vi "ABR3-Initialize.vi"(0 "Params":T1={"CAP or ABR"=enum."ABR", "Stimulus"={"Ear"=enum."Left", "Waveform"=enum."TONE PIP", "Frequency (kHz)"="", "Rep rate (/sec)"=30.0, "Alternate Polarity"=FALSE, "WavFiles"="", "Level (dB SPL)"=30.0, "WavFolder"=path "", "Chirp"={"Type"=enum."AN latency-corrected", "Duration (ms)"=0.0, "Fmin (kHz)"=0.0, "Fmax (kHz)"=0.0, "precompensate"=FALSE}, "Noise"={"Seed"=0, "InvFilt"=FALSE, "AWeight"=FALSE, "afile"=path "", "Filter"={"Type"=enum."Lowpass", "CF (kHz)"=0.0, "BW (kHz)"=0.0, "Cascade"=FALSE, "Quadrature"=FALSE, "Scale Factor"=0.0, "Stages"=[], "Class"=enum."Elliptic", "Order"=0, "BWUnits"=enum."Linear"}}}, "Masker"={"Filter"={"Type"=enum."Lowpass", "CF (kHz)"=0.0, "BW (kHz)"=0.0, "Cascade"=FALSE, "Quadrature"=FALSE, "Scale Factor"=0.0, "Stages"=[], "Class"=enum."Elliptic", "Order"=0, "BWUnits"=enum."Linear"}, "Use masker"=FALSE, "Level"={"Level"=0.0, "Units"=enum."dB atten", "Max"=0.0, "Multiplier"=0.0, "Cal File"=path "", "Cal"={"Freq (Hz)"=[], "Mag (dB SPL)"=[], "Phase (deg)"=[]}}, "Audiogram Comp"=FALSE, "Audiogram File"=path "", "InvFilt"=FALSE}, "Sequence"={"Start (dB)"=20, "Stop (dB)"=80, "Step (dB)"=5, "Var"=enum."Signal", "Order"=enum."Sequential"}, "Controls"={"on"=FALSE, "value"=0.0, "spacing"=0}, "Response"={"Gain"=10000, "Averages"=512, "Window (ms)"=8.5, "Thr Fast Steps"=8.5, "AI Fs"=0.0}, "Hidden"={"AO Samp Rate Hz"=100000.0, "Duration (ms)"=5.0, "Ramp (ms)"=0.5, "Click width (us)"=0.0}} {"Response"."Thr Fast Steps" format="%.2f"; "Response"."Window (ms)" format="%.2f"; "Sequence"."Start (dB)" step=5}, 1 "State":T39, 2 "Resume":bool, 11 "error in (no error)":errorcluster, 12 "Analysis In":T12) -> (3 "Runtime":T37={"Ceiling"=0.0, "Threshold"=0.0, "Crossed?"=FALSE, "Step"=0, "Stop"=0, "Avgs"=0, "Level"=0.0, "AI Npts"=0, "Doubled?"=FALSE, "Gain"=0.0, "NWindowPts"=0, "dt"=0.0, "Cal"=path "", "Freq"=0.0, "AO Channels"=[], "AltPol"=FALSE, "AO Npts"=0, "AO Fs"=0.0, "Start"=0, "Stop max"=0, "Ear"=enum."Right", "Waveform"=enum."TONE PIP", "RepRate"=0.0, "CAP or ABR"=1, "LMasker"=0.0, "SeqVar"=enum."Signal Level", "Reps/buffer"=0, "Avg Mode"=enum."Neural/CM", "Wav"=path "", "Order"=enum."Sequential", "Levels"=[], "ControlVal"=0.0, "innerIndex"=0, "indexStep"=0} {"CAP or ABR" items=["CAP", "ABR"]}, 4 "Stimulus out":T14[](xcontrol), 8 "outerVals":cluster{"wavfile":path, "freq":dbl}[](array[cluster]), 14 "Analysis":T12, 15 "error out":errorcluster)   [LabVIEW 2020]
uses:
  epl-vi-lib/Utility VIs/Type Defs/Left-Right ring.ctl
  CFTS Main Panel SubVIs/CFTS-Experiment State.ctl
  epl-vi-lib/Signal Synthesis VIs/Controls/Advanced Filter XCtl/Advanced Filter XCtl.xctl
  epl-vi-lib/Signal Synthesis VIs/Controls/Level XCtl/Level XCtl.xctl
  epl-vi-lib/Signal Synthesis VIs/Controls/Multichannel (Full)/Multichannel (Full).xctl
  TypeDefs/ABR3-Stimulus.ctl
  TypeDefs/ABR3-Response.ctl
  TypeDefs/ABR3-Seq Var Enum.ctl
  TypeDefs/ABR3-Sequence Spec.ctl
  TypeDefs/ABR3-Masker Spec.ctl
  TypeDefs/ABR-Waveform Enum.ctl
  TypeDefs/ABR3-Controls.ctl
  TypeDefs/ABR3-Parameters.ctl
  TypeDefs/ABR3-Hidden Params.ctl
  TypeDefs/ABR3-Runtime Data.ctl
  TypeDefs/ABR3-Analysis State.ctl
  Threshold Estimation VIs/ABR3-Threshold Estimation Result.ctl
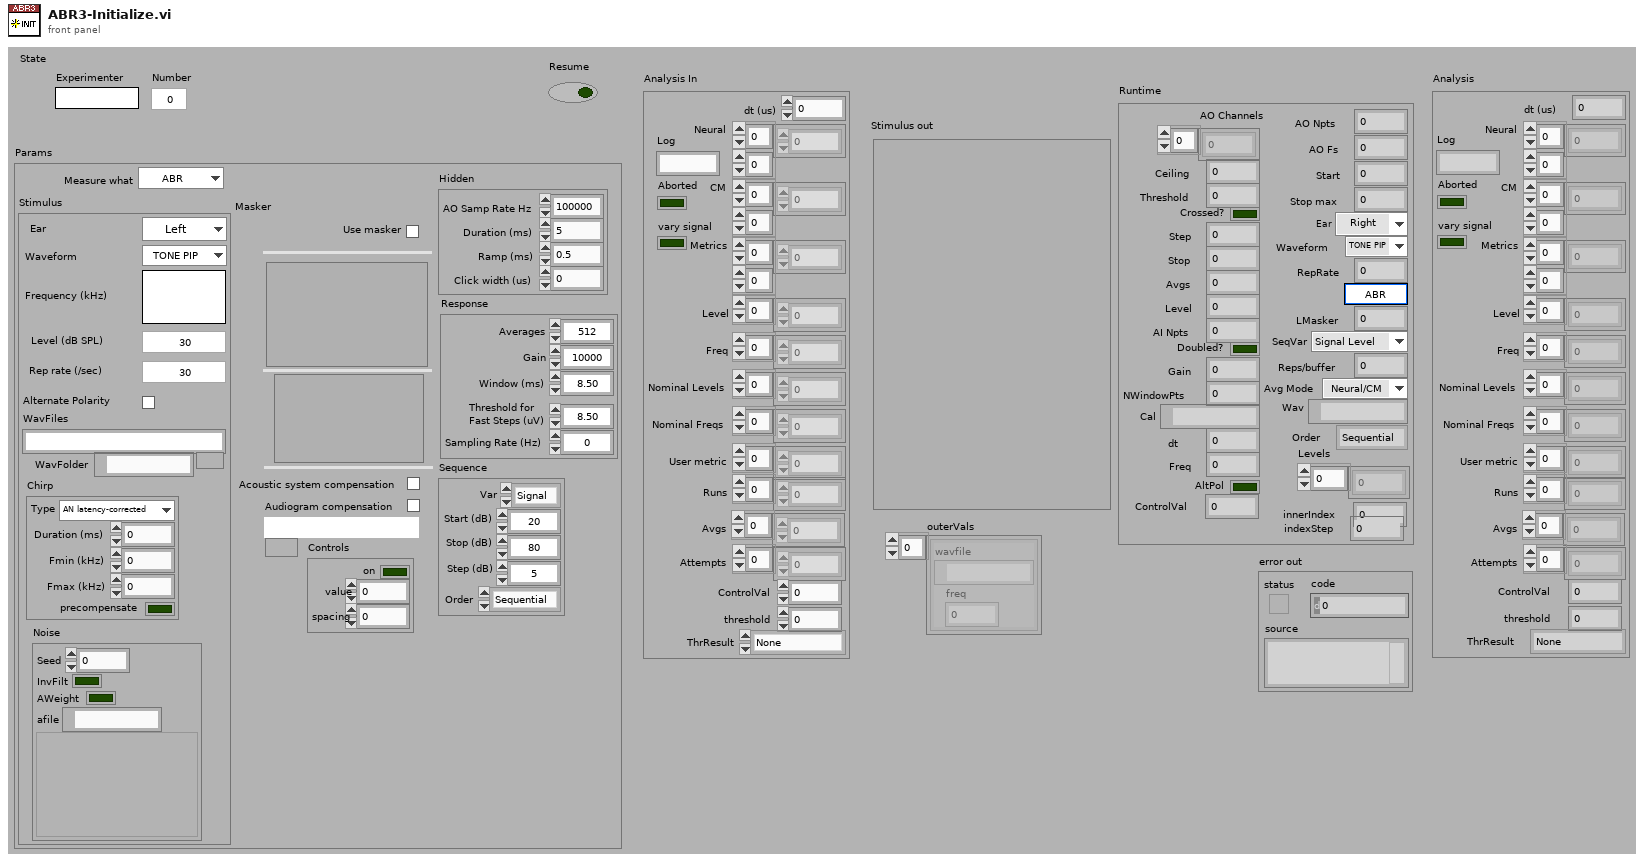
[diagram p1: front panel]
types:
  T1 = typedef "ABR3-Parameters.ctl" = cluster{"CAP or ABR":enum16{"CAP", "ABR"}, "Stimulus":T2, "Masker":T6, "Sequence":T8, "Controls":T9, "Response":T10, "Hidden":T11}
  T2 = typedef "ABR3-Stimulus.ctl" = cluster{"Ear":T3, "Waveform":T4, "Frequency (kHz)":string, "Rep rate (/sec)":dbl, "Alternate Polarity":bool, "WavFiles":string, "Level (dB SPL)":dbl, "WavFolder":path, "Chirp":cluster{"Type":enum16{"AN latency-corrected", "Arbitrary"}, "Duration (ms)":dbl, "Fmin (kHz)":dbl, "Fmax (kHz)":dbl, "precompensate":bool}, "Noise":cluster{"Seed":i32, "InvFilt":bool, "AWeight":bool, "afile":path, "Filter":cluster{"Type":enum16{"Lowpass", "Highpass", "Bandpass", "Bandstop", "OFF"}, "CF (kHz)":dbl, "BW (kHz)":dbl, "Cascade":bool, "Quadrature":bool, "Scale Factor":dbl, "Stages":cluster{"IIR Filter":cluster{"filter structure":enum32{"IIR 2nd Order", "IIR 4th Order"}, "Reverse Coefficients":dbl[], "Forward Coefficients":dbl[]}, "State":dbl[]}[], "Class":enum16{"Elliptic", "Butterworth"}, "Order":i32, "BWUnits":T5}}}
  T3 = typedef "Left-Right ring.ctl" = enum16{"Right", "Left"}
  T4 = typedef "ABR-Waveform Enum.ctl" = enum16{"TONE PIP", "CLICK", "FILE", "CHIRP", "NOISE", "VERHULST"}
  T5 = typedef "Filter-Bandwidth Units.ctl" = enum16{"Linear", "Octaves", "Min-Max"}
  T6 = typedef "ABR3-Masker Spec.ctl" = cluster{"Filter":cluster{"Type":enum16{"Lowpass", "Highpass", "Bandpass", "Bandstop", "OFF"}, "CF (kHz)":dbl, "BW (kHz)":dbl, "Cascade":bool, "Quadrature":bool, "Scale Factor":dbl, "Stages":cluster{"IIR Filter":cluster{"filter structure":enum32{"IIR 2nd Order", "IIR 4th Order"}, "Reverse Coefficients":dbl[], "Forward Coefficients":dbl[]}, "State":dbl[]}[], "Class":enum16{"Elliptic", "Butterworth"}, "Order":i32, "BWUnits":T5}, "Use masker":bool, "Level":cluster{"Level":dbl, "Units":T7, "Max":dbl, "Multiplier":dbl, "Cal File":path, "Cal":cluster{"Freq (Hz)":dbl[], "Mag (dB SPL)":dbl[], "Phase (deg)":dbl[]}}, "Audiogram Comp":bool, "Audiogram File":path, "InvFilt":bool}
  T7 = typedef "Level Units.ctl" = enum16{"dB atten", "dB SPL", "dB re 1 Vrms", "dB V/Hz½", "mW", "dB HL", "Volts", "dB mW"}
  T8 = typedef "ABR3-Sequence Spec.ctl" = cluster{"Start (dB)":i32, "Stop (dB)":i32, "Step (dB)":i32, "Var":enum16{"Signal", "Masker"}, "Order":enum16{"Sequential", "Random"}}
  T9 = typedef "ABR3-Controls.ctl" = cluster{"on":bool, "value":dbl, "spacing":i32}
  T10 = typedef "ABR3-Response.ctl" = cluster{"Gain":i32, "Averages":i32, "Window (ms)":sgl, "Thr Fast Steps":sgl, "AI Fs":dbl}
  T11 = typedef "ABR3-Hidden Params.ctl" = cluster{"AO Samp Rate Hz":dbl, "Duration (ms)":dbl, "Ramp (ms)":dbl, "Click width (us)":dbl}
  T12 = typedef "ABR3-Analysis State.ctl" = cluster{"dt (us)":dbl, "Neural":dbl[][], "CM":dbl[][], "Metrics":dbl[][], "Level":dbl[], "Freq":dbl[], "Nominal Levels":dbl[], "Nominal Freqs":dbl[], "User metric":dbl[], "Runs":i32[], "Avgs":i32[], "Attempts":i32[], "Log":string, "Aborted":bool, "ControlVal":dbl, "threshold":dbl, "vary signal":bool, "ThrResult":T13}
  T13 = typedef "ABR3-Threshold Estimation Result.ctl" = enum16{"None", "Power", "Sigmoid", "Power (noisy)", "Suprathreshold", "Invalid"}
  T14 = typedef "Stimulus Channel (Full).xctl/Full Stimulus Channel Data.ctl" = cluster{"Waveform":T15, "Filter":T32, "Burst":T33, "Level":T34, "Name":string, "Advanced":T35, "SAM":T36}
  T15 = typedef "Waveform XCtl.xctl/Waveform Data.ctl" = cluster{"Type":T16, "Tone":T17, "Pulse Train":T18, "Noise":T21, "File":T22, "FMSweep":T23, "Chirp Train":T24, "Complex Tone":cluster{"Params":T26, "Data":T28}, "Moving Ripple":T29}
  T16 = typedef "Waveform Enum.ctl" = enum16{"OFF", "Tone", "Noise", "Pulse Train", "File", "FM Sweep", "Chirp Train", "Complex Tone", "FM Tone", "Moving Ripple"}
  T17 = typedef "Tone Params.ctl" = cluster{"Frequency (kHz)":dbl, "Last Freq":dbl, "Last Phase":dbl}
  T18 = typedef "Pulse Train Params.ctl" = cluster{"Pulse width (us)":dbl, "Pulse rate (Hz)":dbl, "Gap (ms)":dbl, "Polarity":T19, "PT State":T20, "Asynch":bool}
  T19 = typedef "Pulse Polarity.ctl" = enum16{"POS", "NEG", "POS-NEG", "NEG-POS"}
  T20 = typedef "PT-Continuous State.ctl" = cluster{"Template":dbl[], "Nperiod":i32, "Index":i32, "Pulse Rate (Hz)":dbl, "Phase (cycles)":dbl, "Noff":i32}
  T21 = typedef "Noise Params.ctl" = cluster{"InvFilt":bool, "Noise":dbl[], "CurPt":i32, "Aweight":bool, "Seed":i32, "afile":path}
  T22 = typedef "StimFile-Params.ctl" = cluster{"Filename":path, "Signal":dbl[], "Channel":i32, "stream":bool, "offset":i32, "nreps":i32, "loops":i32, "Randomize":bool, "order":i32[], "Seed":i32, "Tokens":i32}
  T23 = typedef "FM Sweep Params.ctl" = cluster{"Rate (oct/s)":dbl, "Fmin (Hz)":dbl, "Fmax (Hz)":dbl, "Ramp (ms)":dbl, "Linear":bool}
  T24 = typedef "Chirp Train.ctl" = cluster{"Params":T25, "Data":cluster{"WF":dbl[]}}
  T25 = typedef "Chirp Train Params.ctl" = cluster{"Fmin (kHz)":dbl, "Fmax (kHz)":dbl, "Compensate":bool, "Duration (ms)":dbl}
  T26 = typedef "CT-Params.ctl" = cluster{"F0 (Hz)":dbl, "Band":cluster{"Flow (Hz)":dbl, "Fhigh (Hz)":dbl}, "Phase":T27, "Min F0 (Hz)":dbl, "Max F0 (Hz)":dbl, "ContinRandPhase":bool, "Max peak factor":dbl, "Max mod depth":dbl, "MinHarmNum":i32, "MaxHarmNum":i32, "Level Mode":enum16{"per component", "overall rms"}, "% jitter":dbl}
  T27 = typedef "CT-Phase Enum.ctl" = enum16{"Cosine", "Random", "Alternating"}
  T28 = typedef "CT-Runtime Data.ctl" = cluster{"Ncomp":i32, "MinHarm":i32, "Phase":dbl[], "Amplitude":dbl[], "Npts/frame":i32, "Last F0":dbl, "Fmin":dbl, "Fmax":dbl, "Lslope":dbl, "randphase":bool, "overall rms":bool, "fmult":dbl[], "jittered":bool}
  T29 = typedef "Moving Ripple.ctl" = cluster{"Params":T30, "Data":T31}
  T30 = typedef "Moving Ripple.Params.ctl" = cluster{"Fmin":dbl, "Fmax":dbl, "Density":dbl, "Velocity":dbl, "Depth":dbl, "Phase":dbl, "Comp/oct":i32}
  T31 = typedef "Moving Ripple.Data.ctl" = cluster{"Freq":dbl[], "A":dbl[], "phase":dbl[], "Phase":dbl}
  T32 = typedef "Advanced Filter XCtl.xctl/Filter Data.ctl" = cluster{"Type":enum16{"Lowpass", "Highpass", "Bandpass", "Bandstop", "OFF"}, "CF (kHz)":dbl, "BW (kHz)":dbl, "Cascade":bool, "Quadrature":bool, "Scale Factor":dbl, "Stages":cluster{"IIR Filter":cluster{"filter structure":enum32{"IIR 2nd Order", "IIR 4th Order"}, "Reverse Coefficients":dbl[], "Forward Coefficients":dbl[]}, "State":dbl[]}[], "Class":enum16{"Elliptic", "Butterworth"}, "Order":i32, "BWUnits":T5}
  T33 = typedef "Burst Control.xctl/Burst Data.ctl" = cluster{"Active":bool, "Delay (ms)":dbl, "Duration (ms)":dbl, "Ramp (ms)":dbl, "Rate (Hz)":dbl, "Trepeat (ms)":dbl, "Repeat":bool}
  T34 = typedef "Level XCtl.xctl/Level Data.ctl" = cluster{"Level":dbl, "Units":T7, "Max":dbl, "Multiplier":dbl, "Cal File":path, "Cal":cluster{"Freq (Hz)":dbl[], "Mag (dB SPL)":dbl[], "Phase (deg)":dbl[]}}
  T35 = typedef "Advanced Stimulus Options.xctl/Advanced Stimulus Options.ctl" = cluster{"Rep Mask":string, "AltPol":bool, "Var":string, "Expr":string, "Persist":bool}
  T36 = typedef "SAM Params.ctl" = cluster{"Active":bool, "Frequency (Hz)":dbl, "Depth":dbl, "Init Phase (cycles)":dbl, "phase (degrees)":dbl, "Asynch":bool}
  T37 = typedef "ABR3-Runtime Data.ctl" = cluster{"Ceiling":dbl, "Threshold":dbl, "Crossed?":bool, "Step":i32, "Stop":i32, "Avgs":i32, "Level":dbl, "AI Npts":i32, "Doubled?":bool, "Gain":dbl, "NWindowPts":i32, "dt":dbl, "Cal":path, "Freq":dbl, "AO Channels":i32[], "AltPol":bool, "AO Npts":i32, "AO Fs":dbl, "Start":i32, "Stop max":i32, "Ear":T3, "Waveform":T4, "RepRate":dbl, "CAP or ABR":u16, "LMasker":dbl, "SeqVar":T38, "Reps/buffer":i32, "Avg Mode":enum16{"Neural/CM", "ANOW"}, "Wav":path, "Order":enum16{"Sequential", "Random"}, "Levels":dbl[], "ControlVal":dbl, "innerIndex":i32, "indexStep":i32}
  T38 = typedef "ABR3-Seq Var Enum.ctl" = enum16{"Signal Level", "Masker Level"}
  T39 = typedef "CFTS-Experiment State.ctl" = cluster{"Experimenter":string, "Number":u32, "Right":string, "Left":string, "Data Folder":path, "State File":path, "Version Info":string, "End Exposure Time":dbl, "Exposure Duration":string, "Run #":cluster{"CAP":i16, "ABR":i16, "DP":i16, "VsEP":i16, "MeasSeq":i16, "SubSeq":i16, "SFOAE":i16}}
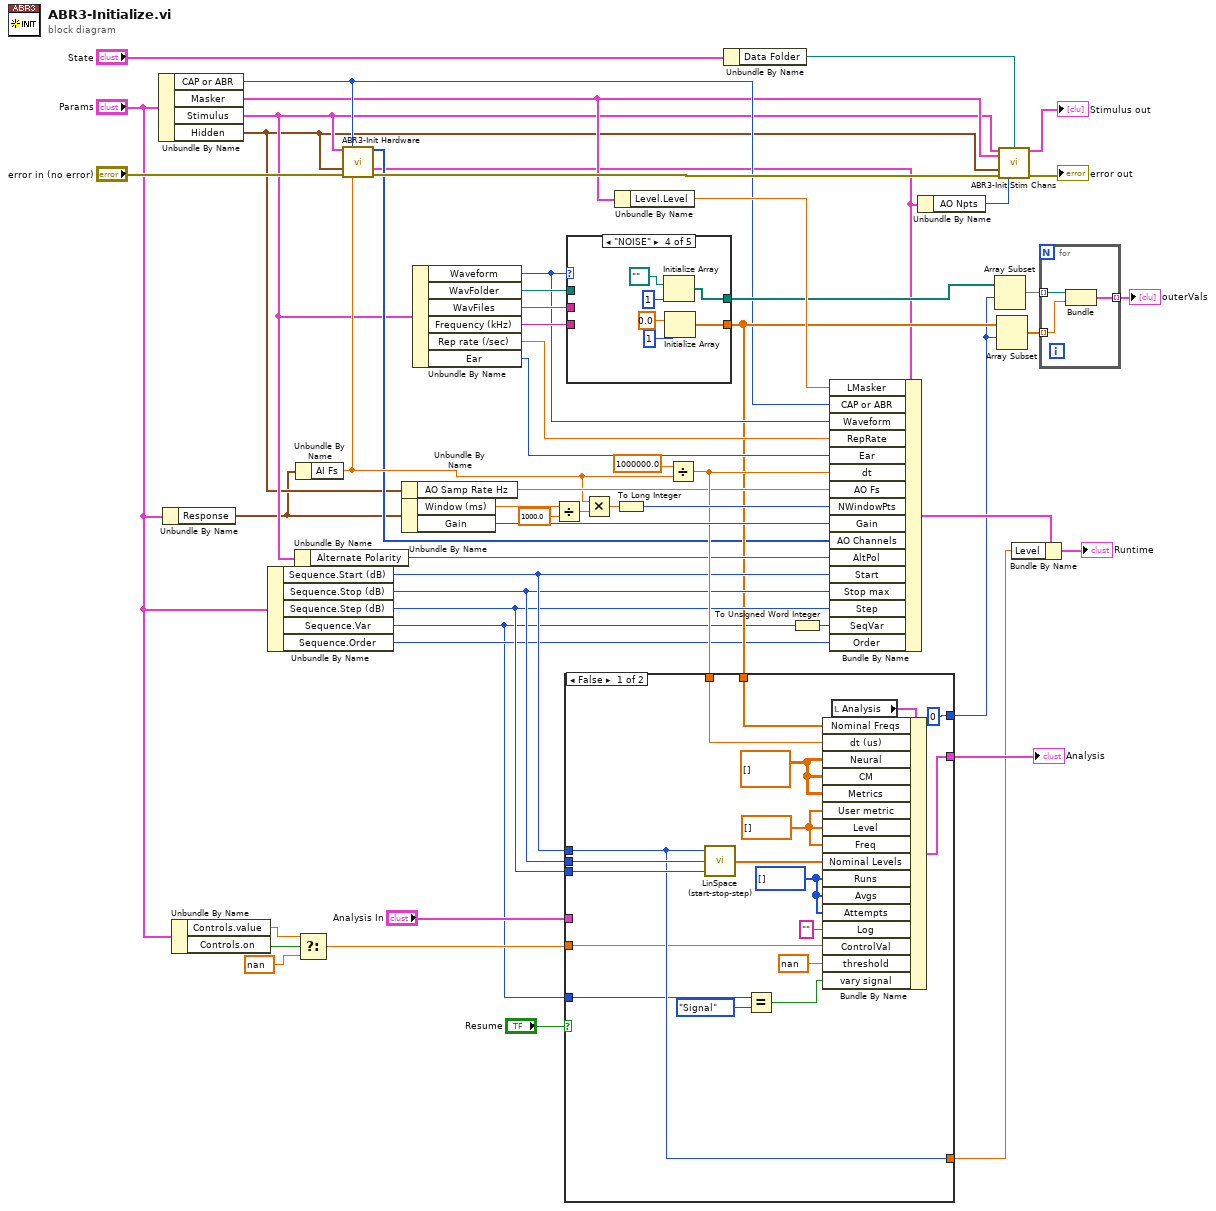
[diagram p0: block diagram]
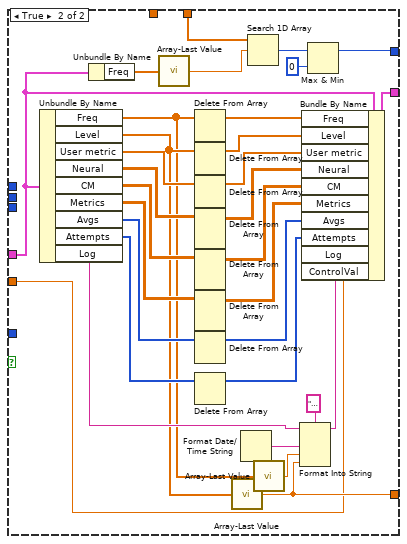
[diagram p2: hidden frame]
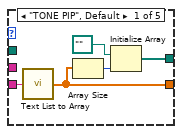
[diagram p3: hidden frame]
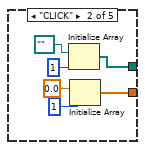
[diagram p4: hidden frame]
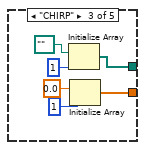
[diagram p5: hidden frame]
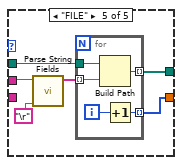
[diagram p6: hidden frame]
diagram:
  n1 = Unbundle By Name("Params") -> ("CAP or ABR"=w17:enum16{"CAP", "ABR"}, "Masker"=w16:T6, "Stimulus"=w15:T2, "Hidden"=w14:T11)
  n2 = Unbundle By Name("Params") -> ("Response"=w1:T10)
  n3 = Unbundle By Name("Params") -> ("Controls.value"=w7:dbl, "Controls.on"=w8:bool)
  n4 = Unbundle By Name("Params") -> ("Sequence.Start (dB)"=w32:i32, "Sequence.Stop (dB)"=w31:i32, "Sequence.Step (dB)"=w30:i32, "Sequence.Var"=w4:enum16{"Signal", "Masker"}, "Sequence.Order"=w10:enum16{"Sequential", "Random"})
  n5 = Unbundle By Name(w15) -> ("Alternate Polarity"=w38:bool)
  n6 = Unbundle By Name(w1) -> ("AI Fs"=w34:dbl)
  n7 = Select(t=w7, s=w8, f=nan) -> (s? t:f=w5:dbl)
  n8 = call "ABR3-Init Hardware.vi"("Stimulus"=w15, "CAP or ABR"=w17, "Hidden"=w14, "error in (no error)"="error in (no error)", "AI Samp Rate Hz"=w34) -> ("AO Channels"=w19:i32[], "Runtime"=w3:T37, "error out"=w42:errorcluster)  [unwired: 7 in, 1 out]
  n9 = Unbundle By Name(w14) -> ("AO Samp Rate Hz"=w39:dbl)
  n10 = Unbundle By Name(w1) -> ("Window (ms)"=w50:sgl, "Gain"=w51:i32)
  n11 = Unbundle By Name(w15) -> ("Waveform"=w27:T4, "WavFolder"=w28:path, "WavFiles"=w29:string, "Frequency (kHz)"=w43:string, "Rep rate (/sec)"=w36:dbl, "Ear"=w35:T3)
  n12 = Divide(x=w50, y=sgl 1000.0) -> (x/y=w48:sgl)
  n13 = case shown="\"NOISE\"" w27 {
    tunnel: w43 -> [w60 _ _ _ _]
    tunnel: [w57 w66 w72 w78 w79] -> w24
    tunnel: w29 -> [_ _ _ _ w83]
    tunnel: w28 -> [_ _ _ _ w84]
    tunnel: [w59 w62 w68 w74 w82] -> w20
    frame "TONE PIP", Default {
      n14 = call "Text List to Array.vi"("text list"=w60) -> ("array"=w57:dbl[])  [unwired: 3 in]
      n15 = Array Size(array=w57) -> (size(s)=w58:i32)
      n16 = Initialize Array(path "", w58) -> (w59:path[])
    }
    frame "CLICK" {
      n17 = Initialize Array(path "", 1 ("dimension size")) -> (w62:path[])
      n18 = Initialize Array(0.0 ("element"), 1 ("dimension size")) -> (w66:dbl[])
    }
    frame "CHIRP" {
      n19 = Initialize Array(path "", 1 ("dimension size")) -> (w68:path[])
      n20 = Initialize Array(0.0 ("element"), 1 ("dimension size")) -> (w72:dbl[])
    }
    frame "NOISE" {
      n21 = Initialize Array(path "", 1 ("dimension size")) -> (w74:path[])
      n22 = Initialize Array(0.0 ("element"), 1 ("dimension size")) -> (w78:dbl[])
    }
    frame "FILE" {
      n23 = call "Parse String Fields.vi"("Separator"="\r", "String"=w83) -> ("Fields"=w80:string[])  [unwired: 8 in, 1 out]
      n24 = for {
        tunnel: w84 -> [w89]
        tunnel: w80 -> [w88] mode=indexing
        tunnel: [w87] -> w82 mode=indexing
        tunnel: [w85] -> w79 mode=indexing
        i -> [w86]
        n25 = Build Path(base path=w89, name or relative path=w88) -> (appended path=w87:path)
        n26 = Increment(x=w86) -> (x+1=w85:i32)
      }
    }
  }
  n27 = Multiply(x=w34, y=w48) -> (x*y=w47:dbl)
  n28 = Unbundle By Name(w16) -> ("Level.Level"=w33:dbl)
  n29 = To Long Integer(number=w47) -> (32bit integer=w46:i32)
  n30 = Divide(x=1000000.0, y=w34) -> (x/y=w44:dbl)
  n31 = case shown="False" "Resume" {
    tunnel: [w106 w131] -> w45
    tunnel: w44 -> [w105 _]
    tunnel: w24 -> [w104 w137]
    tunnel: w32 -> [w95 _]
    tunnel: w31 -> [w102 _]
    tunnel: w30 -> [w101 _]
    tunnel: "Analysis In" -> [_ w132]
    tunnel: [0 ("index of element") w134] -> w23
    tunnel: [w95 w110] -> w21
    tunnel: w5 -> [w94 w108]
    tunnel: w4 -> [w92 _]
    frame False {
      w96 = i32[] [] ("Runs")
      w99 = dbl[] [] ("Level")
      w100 = dbl[][] [] ("Neural")
      n32 = call "LinSpace (start-stop-step).vi"("Step"=w101, "Stop"=w102, "Start"=w95) -> ("Array"=w103:dbl[])  [unwired: 1 in, 1 out]
      n33 = Equal?(x=w92, y=enum16{"Signal", "Masker"}."Signal") -> (x = y?=w90:bool)
      n34 = local read "Analysis"() -> (w107:T12)
      n35 = Bundle By Name(cluster=w107, "Nominal Freqs"=w104, "dt (us)"=w105, "Neural"=w100, "CM"=w100, "Metrics"=w100, "User metric"=w99, "Level"=w99, "Freq"=w99, "Nominal Levels"=w103, "Runs"=w96, "Avgs"=w96, "Attempts"=w96, "Log"="", "ControlVal"=w94, "threshold"=nan, "vary signal"=w90) -> (w106:T12)
    }
    frame True {
      n36 = Unbundle By Name(w132) -> ("Freq"=w109:dbl[], "Level"=w111:dbl[], "User metric"=w130:dbl[], "Neural"=w128:dbl[][], "CM"=w127:dbl[][], "Metrics"=w126:dbl[][], "Avgs"=w122:i32[], "Attempts"=w121:i32[], "Log"=w113:string)
      n37 = Unbundle By Name(w132) -> ("Freq"=w138:dbl[])
      n38 = call "Array-Last Value.vi"("array"=w138) -> ("element"=w136:dbl)
      n39 = Delete From Array(array=w109) -> (array with subset deleted=w118:dbl[])  [unwired: 2 in, 1 out]
      n40 = Delete From Array(array=w111) -> (array with subset deleted=w117:dbl[])  [unwired: 2 in, 1 out]
      n41 = Delete From Array(array=w130) -> (array with subset deleted=w129:dbl[])  [unwired: 2 in, 1 out]
      n42 = Delete From Array(array=w128) -> (array with subset deleted=w125:dbl[][])  [unwired: 3 in, 1 out]
      n43 = Delete From Array(array=w127) -> (array with subset deleted=w123:dbl[][])  [unwired: 3 in, 1 out]
      n44 = Delete From Array(array=w126) -> (array with subset deleted=w124:dbl[][])  [unwired: 3 in, 1 out]
      n45 = Delete From Array(array=w122) -> (array with subset deleted=w120:i32[])  [unwired: 2 in, 1 out]
      n46 = Delete From Array(array=w121) -> (array with subset deleted=w119:i32[])  [unwired: 2 in, 1 out]
      n47 = call "Array-Last Value.vi"("array"=w111) -> ("element"=w110:dbl)
      n48 = Format Date/Time String() -> (date/time string=w114:string)  [unwired: 3 in]
      n49 = Search 1D Array(1D array=w137, element=w136) -> (index of element=w135:i32)  [unwired: 1 in]
      n50 = call "Array-Last Value.vi"("array"=w109) -> ("element"=w115:dbl)
      n51 = Format Into String(format string="Resumed %s on Freq=%#g, Level=%#g\\n", initial string=w113, w114, w115, w110) -> (resulting string=w112:string)  [unwired: 1 in, 1 out]
      n52 = Bundle By Name(cluster=w132, "Freq"=w118, "Level"=w117, "User metric"=w129, "Neural"=w125, "CM"=w123, "Metrics"=w124, "Avgs"=w120, "Attempts"=w119, "Log"=w112, "ControlVal"=w108) -> (w131:T12)
      n53 = Max & Min(x=w135, y=0) -> (max(x,y)=w134:i32)  [unwired: 1 out]
    }
  }
  "Analysis" <- w45
  n54 = Unbundle By Name("State") -> ("Data Folder"=w41:path)
  n55 = To Unsigned Word Integer(number=w4) -> (unsigned 16bit integer=w18:u16)
  n56 = Bundle By Name(cluster=w3, "LMasker"=w33, "CAP or ABR"=w17, "Waveform"=w27, "RepRate"=w36, "Ear"=w35, "dt"=w44, "AO Fs"=w39, "NWindowPts"=w46, "Gain"=w51, "AO Channels"=w19, "AltPol"=w38, "Start"=w32, "Stop max"=w31, "Step"=w30, "SeqVar"=w18, "Order"=w10) -> (w52:T37)
  n57 = Unbundle By Name(w3) -> ("AO Npts"=w2:i32)
  n58 = Array Subset(array=w20, index=w23) -> (w13:path[])  [unwired: 1 in]
  n59 = Array Subset(array=w24, index=w23) -> (w12:dbl[])  [unwired: 1 in]
  n60 = call "ABR3-Init Stim Chans.vi"("Stimulus"=w15, "Masker"=w16, "Data Folder"=w41, "Hidden"=w14, "error in (no error)"=w42, "Npts"=w2) -> ("StimChans"=→"Stimulus out":T14[], "error out"=→"error out":errorcluster)  [unwired: 8 in]
  n61 = Bundle By Name(cluster=w52, "Level"=w21) -> (→"Runtime":T37)
  n62 = for {
    tunnel: w13 -> [w141] mode=indexing
    tunnel: w12 -> [w140] mode=indexing
    tunnel: [w139] -> w11 mode=indexing
    n63 = Bundle("appended path"=w141, "element"=w140) -> (w139:cluster{"appended path":path, "element":dbl})  [unwired: 1 in]
  }
  "outerVals" <- w11
